vi "Assert Number of Initialize and Close Calls.vi"(0 "expected initialize-initialize calls":u32, 5 "expected initialize-attach calls":u32, 7 "expected close-close calls":u32, 9 "expected close-detach calls":u32, 11 "error in":errorcluster) -> (4 "pass":bool, 6 "result":string, 15 "error out":errorcluster)   [LabVIEW 2020, in "MeasurementServerTests.lvlib"]
uses:
  MeasurementServerTests.lvlib
  Fake Instrument/Call Recorder Action.ctl
  Fake Instrument/Fake Instrument.lvclass
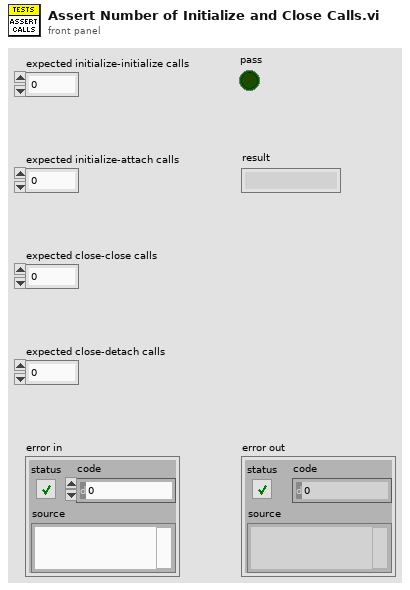
[diagram p1: front panel]
types:
  T1 = typedef "MeasurementServerTests.lvlib/Fake Instrument.lvclass/Call Recorder Action.ctl" = enum16{"Initialize", "Read Values", "Record Initialize-Initialize", "Record Initialize-Attach", "Record Close-Close", "Record Close-Detach"}
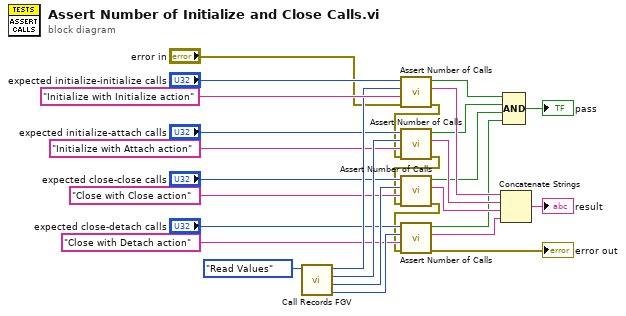
[diagram p0: block diagram]
diagram:
  n1 = call "Call Records FGV.vi"("Call Recorder Action"=Call_Recorder_Action."Read Values") -> ("Close-Detach calls"=w7:u32, "Close-Close calls"=w10:u32, "Initialize-Attach calls"=w13:u32, "Initialize-Initialize calls"=w21:u32)  [unwired: 7 in]
  n2 = call "Assert Number of Calls.vi"("error in"="error in", "name of call"="Initialize with Initialize action" ("input 2"), "actual calls"=w21, "expected calls"="expected initialize-initialize calls") -> ("error out"=w3:errorcluster, "result"=w26:string, "pass"=w24:bool)  [unwired: 5 in]
  n3 = call "Assert Number of Calls.vi"("error in"=w3, "name of call"="Initialize with Attach action" ("input 2"), "actual calls"=w13, "expected calls"="expected initialize-attach calls") -> ("error out"=w2:errorcluster, "result"=w19:string, "pass"=w20:bool)  [unwired: 5 in]
  n4 = call "Assert Number of Calls.vi"("error in"=w2, "name of call"="Close with Close action" ("input 2"), "actual calls"=w10, "expected calls"="expected close-close calls") -> ("error out"=w1:errorcluster, "result"=w17:string, "pass"=w18:bool)  [unwired: 5 in]
  n5 = call "Assert Number of Calls.vi"("error in"=w1, "name of call"="Close with Detach action" ("input 2"), "actual calls"=w7, "expected calls"="expected close-detach calls") -> ("error out"=→"error out":errorcluster, "result"=w15:string, "pass"=w16:bool)  [unwired: 5 in]
  n6 = Concatenate Strings(w26, w19, w17, w15) -> (→"result":string)
  n7 = Compound Arithmetic op=AND(w24, w20, w18, w16) -> (→"pass":bool)
